vi "arithematic operations.vi"() -> ()   [LabVIEW 2025]
panel:
  out "division":dbl
  out "multiplication":dbl
  out "sub":dbl
  out "addtion":dbl
  in  "input b":dbl
  in  "input a":dbl
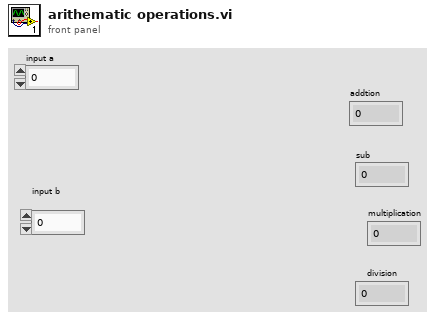
[diagram p1: front panel]
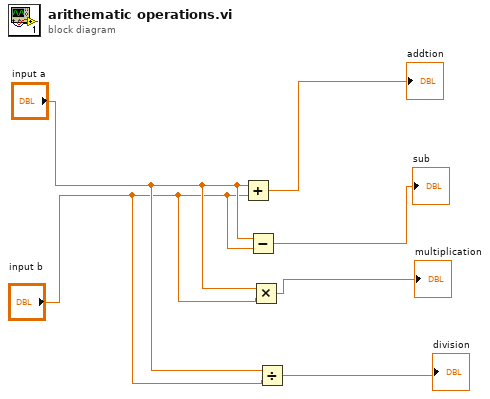
[diagram p0: block diagram]
diagram:
  n1 = Add(x="input a", y="input b") -> (x+y=→"addtion":dbl)
  n2 = Subtract(x="input a", y="input b") -> (x-y=→"sub":dbl)
  n3 = Multiply(x="input a", y="input b") -> (x*y=→"multiplication":dbl)
  n4 = Divide(x="input a", y="input b") -> (x/y=→"division":dbl)
